vi "FIB realtime imaging PXIe-6124.vi"(0 "HW Config":T4={"FIB X coil"="FIB/ao0", "FIB Y coil"="FIB/ao1", "Beam blank"="FIB/port0/line0", "Ext Scan"="FIB/port0/line1", "Detector"="FIB/ai1", "Shutter Drive"="PXI1Slot2/ao0"}, 1 "Options":T3 {"Scan mode" items=["Raster", "Serpentine"]; "Det" items=["Detector A", "Detector B"]}, 2 "Single scan":bool, 3 "Scan Para":T2={"X resolution"=512, "Z resolution"=512, "X center"=0.0, "Z center"=0.0, "X size (V)"=10.0, "Z size (V)"=10.0, "Frame line rampdown ratio"=-0.1, "Scan rate (Hz)"=2000000, "Oversampling"=2} {"Frame line rampdown ratio" min=-1.0 max=1.0 step=0.05 format="%.2g"; "Scan rate (Hz)" max=4000000 format="%#.6p"}, 4 "As subVi":bool, 5 "COM port":refnum<visa-resource-name>="COM1", 6 "ActiveX Container":refnum<k7>(container)) -> (7 "Info & Status":T1={"Actual scan rate"=2000000.0, "X resolution with rampdown"=552, "Actual sample rate"=4000000.0, "Fetch backlog"=664878.0, "Total scan points"=276000, "Frame rate (/s)"=7} {"Fetch backlog" format="%#_6p"; "Actual sample rate" format="%#_6p"; "Actual scan rate" format="%#_4p"}, 10 "error out":errorcluster)   [LabVIEW 2018]
uses:
  <vilib>/DAQmx/write.llb/DAQmx Write (Analog 1D DBL NChan 1Samp).vi
  <vilib>/DAQmx/write.llb/DAQmx Write (Digital Wfm 1Chan NSamp).vi
  <vilib>/DAQmx/write.llb/DAQmx Write (Analog 2D DBL NChan NSamp).vi
  <vilib>/DAQmx/read.llb/DAQmx Read (Raw 1D I16).vi
  <vilib>/Analysis/2dsp.llb/Decimate (single shot, DBL).vi
  <vilib>/DAQmx/create/channels.llb/DAQmx Create Channel (AI-Voltage-Basic).vi
  <vilib>/DAQmx/create/channels.llb/DAQmx Create Channel (AO-Voltage-Basic).vi
  <vilib>/DAQmx/miscellaneous.llb/DAQmx Fill In Error Info.vi
  <vilib>/Waveform/DWDTOps.llb/DWDT Invert Digital.vi
  <vilib>/DAQmx/configure/timing.llb/DAQmx Timing (Sample Clock).vi
  <vilib>/DAQmx/create/channels.llb/DAQmx Create Channel (DO-Digital Output).vi
  <vilib>/DAQmx/create/channels.llb/DAQmx Create Channel (CO-Pulse Generation-Frequency).vi
  <vilib>/DAQmx/configure/trigger.llb/DAQmx Start Trigger (Digital Edge).vi
  <vilib>/Waveform/DWDTOps.llb/DWDT Uncompress Digital.vi
  <vilib>/Waveform/DWDTOps.llb/Digital Pattern Generator (Single Value).vi
  <vilib>/Analysis/NI_AALPro.lvlib
  <resource>/objmgr/daqmx.rc
panel:
  in  "Spot":bool
  out "Image shift":u32
  out "AI SampleClk.MaxRate":dbl
  in  "Sweep enabled":bool
  in  "Focus (V)":dbl min=-10.0 max=10.0 step=0.1 format="%.3g"
  in  "Sweep rate (Hz)":dbl=0.5 min=0.01 step=0.1 format="%0.2f"
  in  "Level #":u8
  in  "Sweep direction":bool
  in  "Angle (V)":dbl min=-10.0 max=10.0 step=0.1 format="%.3g"
  in  "Position (V)":dbl min=-10.0 max=10.0 step=0.1 format="%.3g"
  in  "Imbalance (V)":dbl min=-10.0 max=10.0 step=0.1 format="%.3f"
  out "Shutter Drive":tag
  out "Low blanked":bool
  in  "Machine Type":u8(ring) items=["Feiss", "NVision", "Jeiss"]
  out "Ext scan":tag
  out "Detector":tag="PXI1Slot7/ai0"
  out "FIB Y coil":tag="PXI1Slot7/ao1"
  out "FIB X coil":tag="PXI1Slot7/ao0"
  in  "Beam blanked":bool
  out "Beam blank":tag="PXI1Slot7/port0/line0"
  out "Oversampling":u16=2
  out "Scan rate (Hz)":u32=2000000
  out "Frame line rampdown ratio":dbl=0.1
  out "Y end":dbl=1.0
  out "X end":dbl=1.0
  out "Y start":dbl=-1.0
  out "X start":dbl=-1.0
  out "Y resolution":u32=500
  out "X resolution":u32=500
  out "Flip z":bool
  out "Flip x":bool
  out "Scan mode":u16
  out "Live image":i16[][](graph)
  in  "stop":bool=TRUE
  # "Flip"
  # "Scan coils"
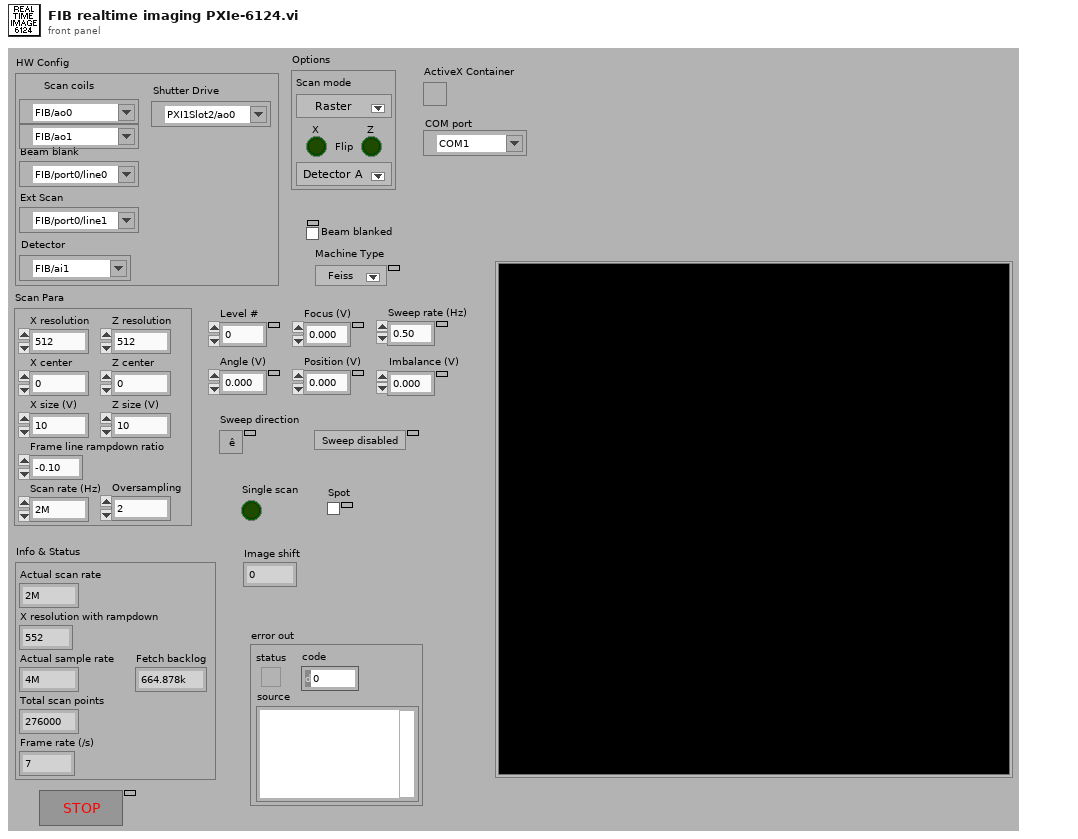
[diagram p1: front panel]
types:
  T1 = cluster{"Actual scan rate":dbl, "X resolution with rampdown":i32, "Actual sample rate":dbl, "Fetch backlog":dbl, "Total scan points":i32, "Frame rate (/s)":u32}
  T2 = cluster{"X resolution":u32, "Z resolution":u32, "X center":dbl, "Z center":dbl, "X size (V)":dbl, "Z size (V)":dbl, "Frame line rampdown ratio":dbl, "Scan rate (Hz)":u32, "Oversampling":u16}
  T3 = cluster{"Scan mode":u16, "Flip x":bool, "Flip z":bool, "Det":u16}
  T4 = cluster{"FIB X coil":tag, "FIB Y coil":tag, "Beam blank":tag, "Ext Scan":tag, "Detector":tag, "Shutter Drive":tag}
  T5 = enum16{"SEM", "FIB", "Milling", "SEM + FIB", "Mill + SEM", "SEM Drift Correction", "FIB Drift Correction", "No Beam", "External", "External + SEM"}
  T6 = enum16{"SEM", "FIB", "Mill", "SEM + FIB", "Mill + SEM", "Drift SEM", "Drift FIB", "None", "Ext", "Ext + SEM"}
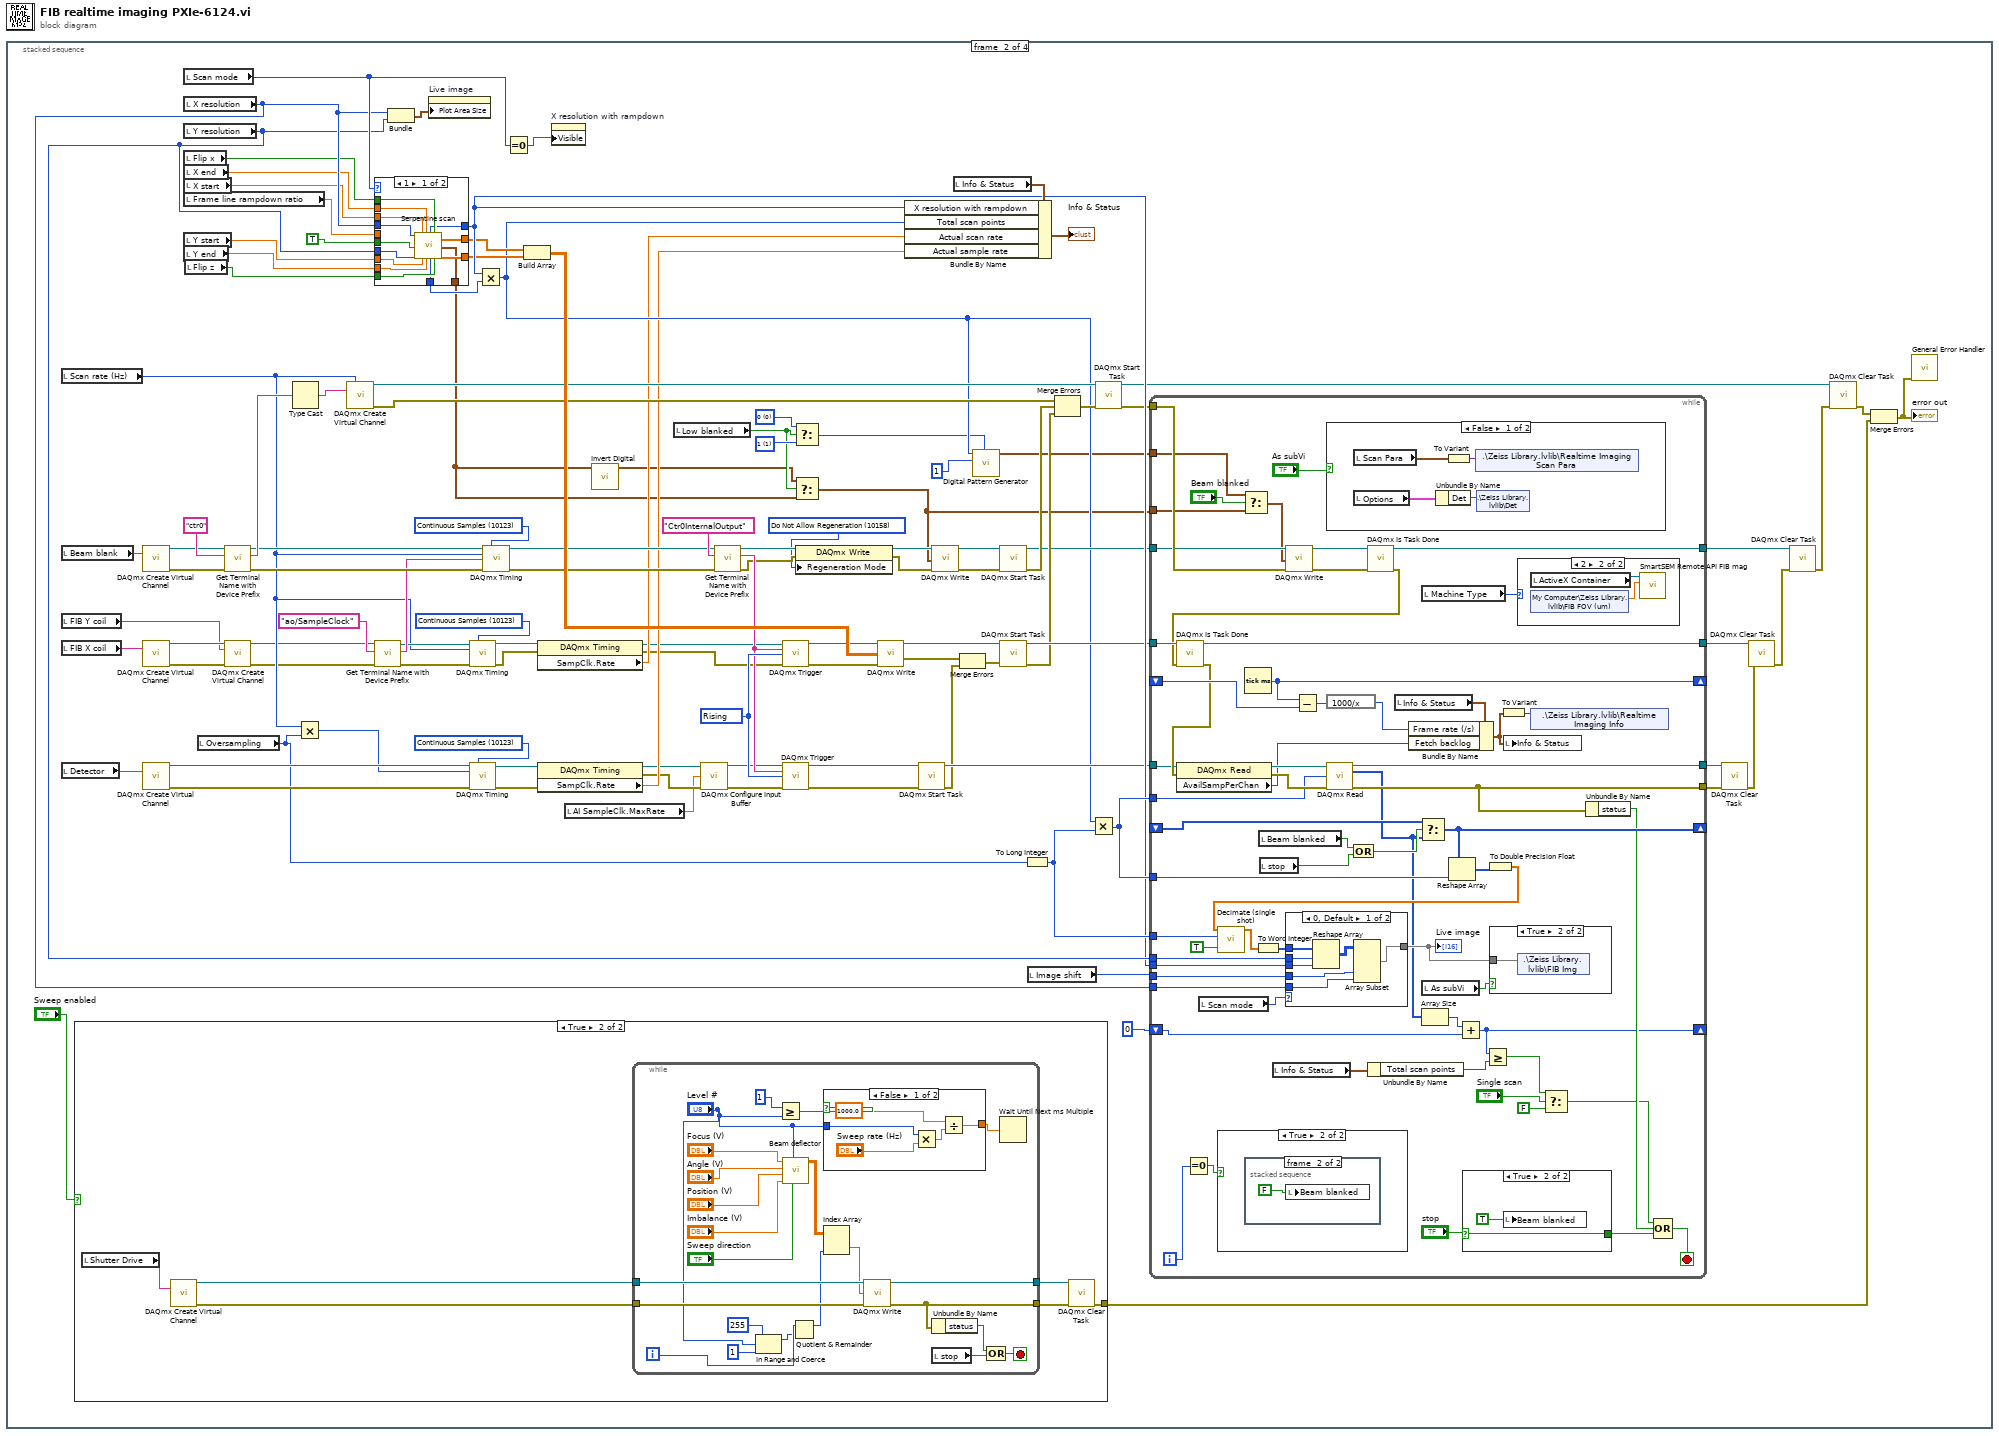
[diagram p0: block diagram]
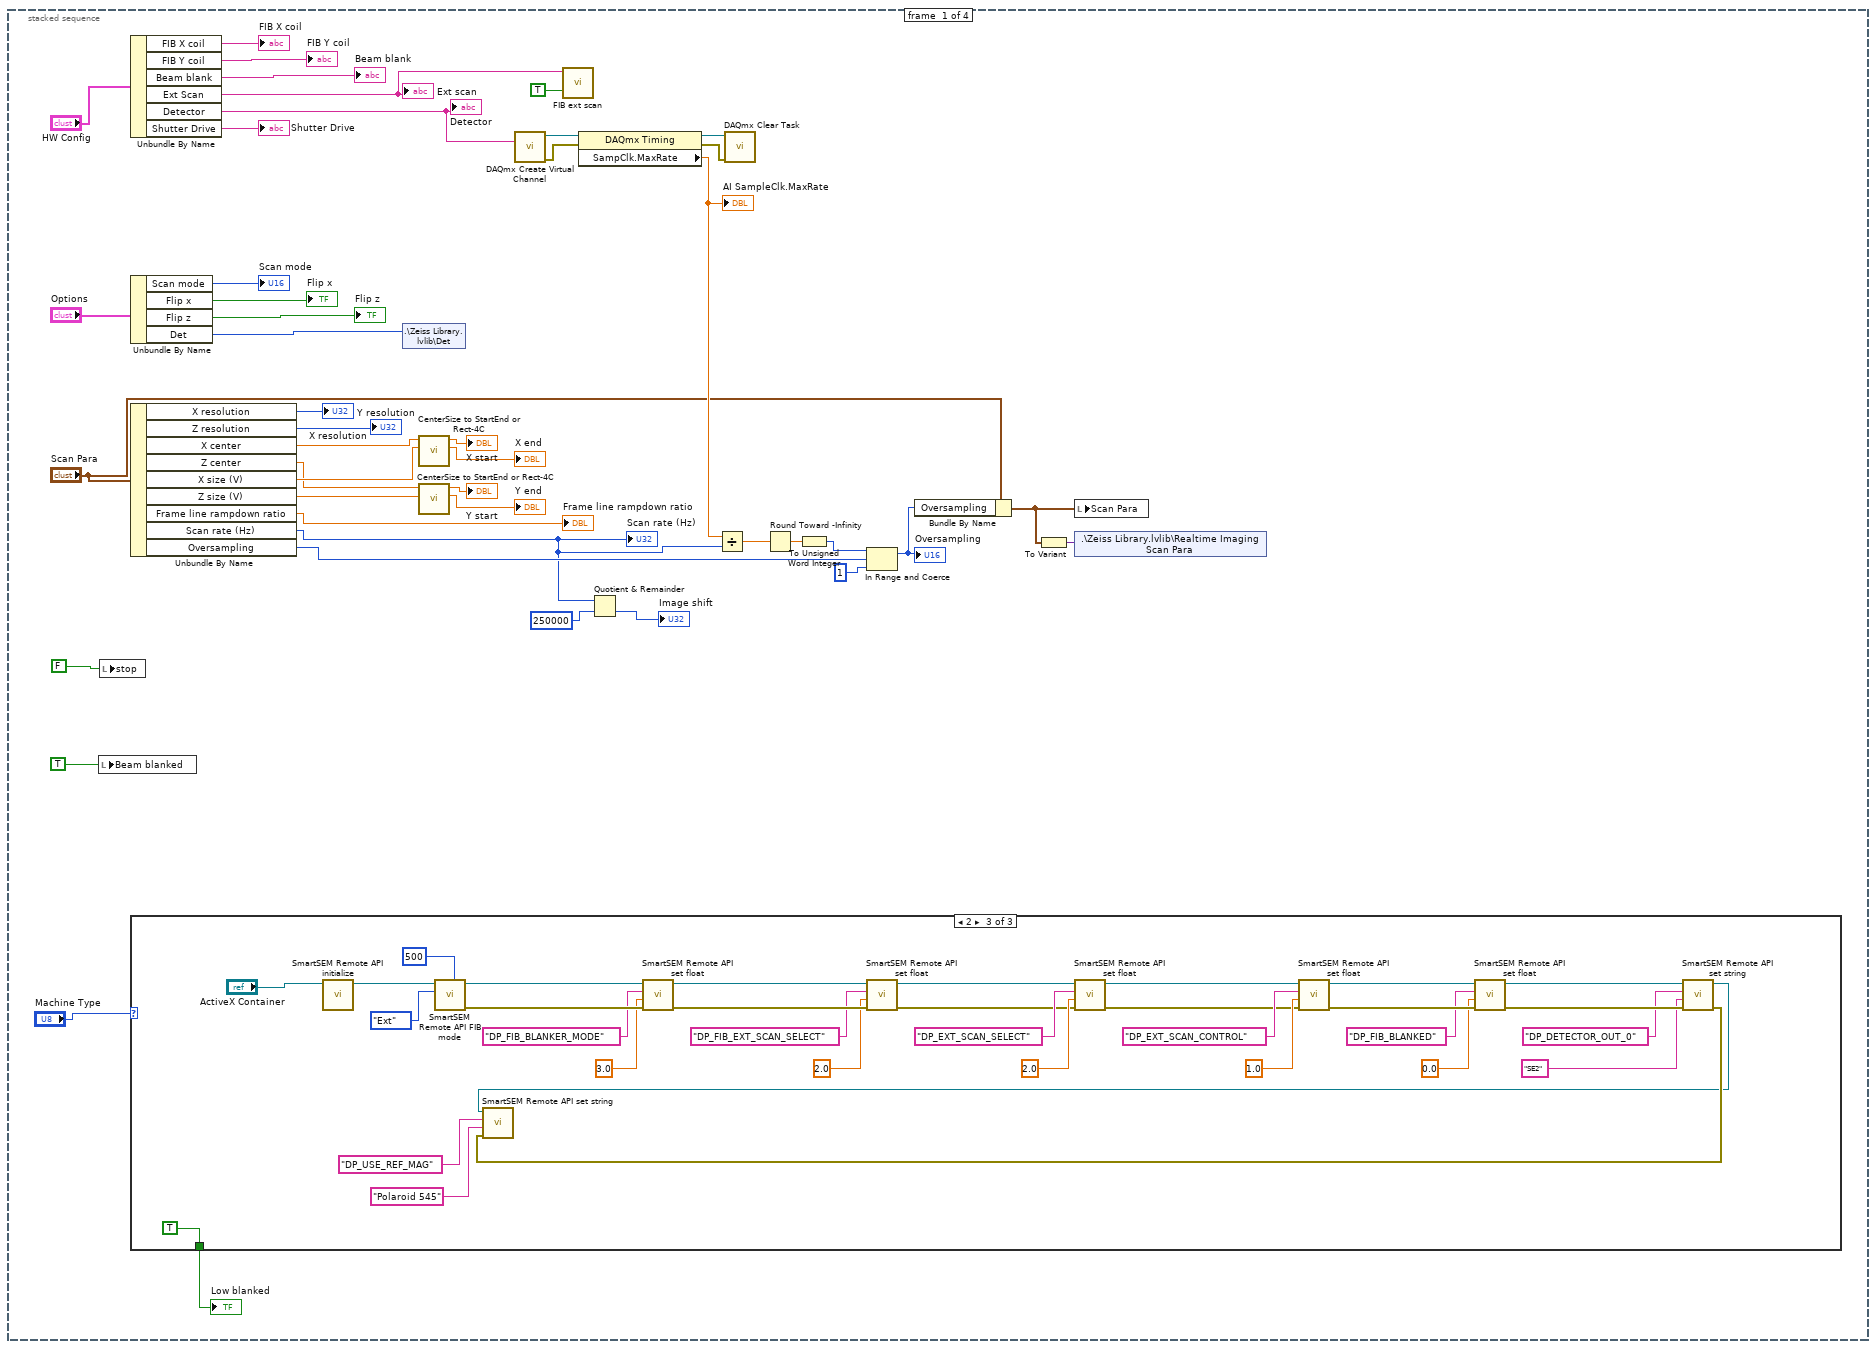
[diagram p2: hidden frame]
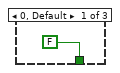
[diagram p3: hidden frame]
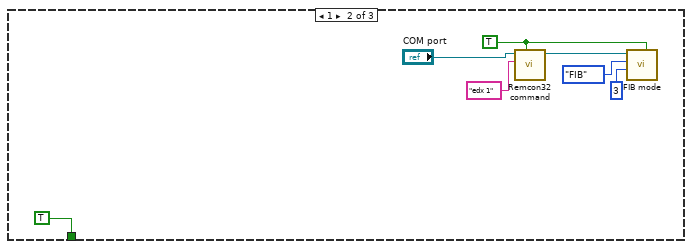
[diagram p4: hidden frame]
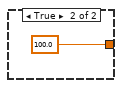
[diagram p6: hidden frame]
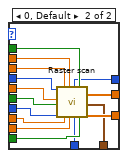
[diagram p7: hidden frame]
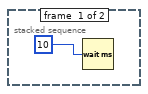
[diagram p11: hidden frame]
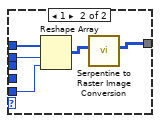
[diagram p14: hidden frame]
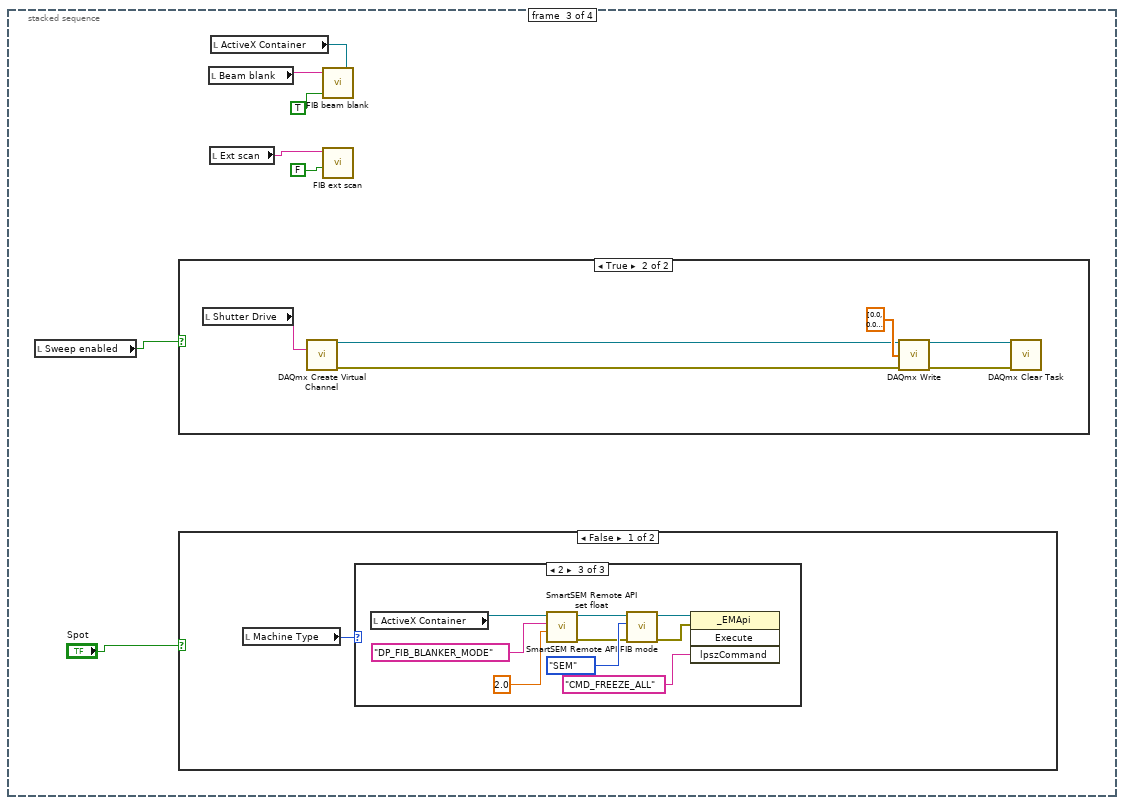
[diagram p15: hidden frame]
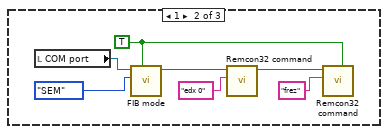
[diagram p17: hidden frame]
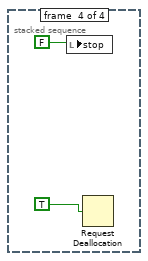
[diagram p20: hidden frame]
diagram:
  n1 = stacked-sequence {
    frame #0 {
      n2 = local write "Beam blanked"(TRUE ("Beam blanked")) -> ()
      n3 = local write "stop"(FALSE ("stop")) -> ()
      n4 = Unbundle By Name("HW Config") -> ("FIB X coil"=→"FIB X coil":tag, "FIB Y coil"=→"FIB Y coil":tag, "Beam blank"=→"Beam blank":tag, "Ext Scan"=w23:tag, "Detector"=w16:tag, "Shutter Drive"=→"Shutter Drive":tag)
      "Detector" <- w16
      "Ext scan" <- w23
      n5 = Unbundle By Name("Options") -> ("Scan mode"=→"Scan mode":u16, "Flip x"=→"Flip x":bool, "Flip z"=→"Flip z":bool, "Det"=w37:u16)
      n6 = Unbundle By Name("Scan Para") -> ("X resolution"=→"X resolution":u32, "Z resolution"=→"Y resolution":u32, "X center"=w34:dbl, "Z center"=w30:dbl, "X size (V)"=w33:dbl, "Z size (V)"=w29:dbl, "Frame line rampdown ratio"=→"Frame line rampdown ratio":dbl, "Scan rate (Hz)"=w5:u32, "Oversampling"=w15:u16)
      "Scan rate (Hz)" <- w5
      n7 = case shown="2" "Machine Type" {
        tunnel: [FALSE ("Beam blanked") TRUE ("Beam blanked") TRUE ("Beam blanked")] -> w21
        frame 0, Default {
        }
        frame 1 {
          w50 = TRUE ("Close session")
          n8 = call "Remcon32 command.vi"("Initialization"=w50, "SEM command"="edx 1", "COM port in"="COM port") -> ("COM port out"=w49:refnum<visa-resource-name>)  [unwired: 5 in, 3 out]
          n9 = call "FIB mode.vi"("Close session"=w50, "Iterations"=u32 3, "FIB mode"=T5."FIB", "COM port in"=w49) -> ()  [unwired: 6 in, 2 out]
        }
        frame 2 {
          n10 = call "SmartSEM Remote API initialize.vi"("ActiveX Container"="ActiveX Container") -> ("reference out"=w58:refnum<k7>)  [unwired: 9 in, 1 out]
          n11 = call "SmartSEM Remote API FIB mode.vi"("Wait (ms)"=u32 500, "FIB mode"=T6."Ext", "ActiveX Container"=w58) -> ("error out"=w83:errorcluster, "reference out"=w84:refnum<k7>)  [unwired: 7 in]
          n12 = call "SmartSEM Remote API set float.vi"("error in"=w83, "vValue"=sgl 3.0, "lpszParam"="DP_FIB_BLANKER_MODE", "ActiveX Container"=w84) -> ("error out"=w79:errorcluster, "reference out"=w80:refnum<k7>)  [unwired: 6 in]
          n13 = call "SmartSEM Remote API set float.vi"("error in"=w79, "vValue"=sgl 2.0, "lpszParam"="DP_FIB_EXT_SCAN_SELECT" ("lpszCommand"), "ActiveX Container"=w80) -> ("error out"=w57:errorcluster, "reference out"=w55:refnum<k7>)  [unwired: 6 in]
          n14 = call "SmartSEM Remote API set float.vi"("error in"=w57, "vValue"=sgl 2.0, "lpszParam"="DP_EXT_SCAN_SELECT" ("lpszCommand"), "ActiveX Container"=w55) -> ("error out"=w56:errorcluster, "reference out"=w54:refnum<k7>)  [unwired: 6 in]
          n15 = call "SmartSEM Remote API set float.vi"("error in"=w56, "vValue"=sgl 1.0, "lpszParam"="DP_EXT_SCAN_CONTROL" ("lpszCommand"), "ActiveX Container"=w54) -> ("error out"=w73:errorcluster, "reference out"=w74:refnum<k7>)  [unwired: 6 in]
          n16 = call "SmartSEM Remote API set float.vi"("error in"=w73, "vValue"=sgl 0.0, "lpszParam"="DP_FIB_BLANKED", "ActiveX Container"=w74) -> ("error out"=w69:errorcluster, "reference out"=w70:refnum<k7>)  [unwired: 6 in]
          n17 = call "SmartSEM Remote API set string.vi"("error in"=w69, "vValue"="SE2" ("Det A Type"), "lpszParam"="DP_DETECTOR_OUT_0", "ActiveX Container"=w70) -> ("error out"=w61:errorcluster, "reference out"=w60:refnum<k7>)  [unwired: 6 in]
          n18 = call "SmartSEM Remote API set string.vi"("error in"=w61, "vValue"="Polaroid 545" ("lpszParam"), "lpszParam"="DP_USE_REF_MAG", "ActiveX Container"=w60) -> ()  [unwired: 6 in, 2 out]
        }
      }
      "Low blanked" <- w21
      n19 = shared-variable ".\\Zeiss Library.lvlib\\Det"(w37) -> ()  [unwired: 1 in, 1 out]
      n20 = call "CenterSize to StartEnd or Rect-4C.vi"("Size"=w33, "Center"=w34) -> ("End"=→"X end":dbl, "Start"=→"X start":dbl)  [unwired: 3 in, 1 out]
      n21 = call "CenterSize to StartEnd or Rect-4C.vi"("Size"=w29, "Center"=w30) -> ("End"=→"Y end":dbl, "Start"=→"Y start":dbl)  [unwired: 3 in, 1 out]
      n22 = call-poly <vilib>:"DAQmx Create Virtual Channel.vi"("physical channels"=w16) -> ("task out"=w18:refnum<k21>, "error out"=w20:errorcluster)  [unwired: 8 in, 5 out]
      n23 = call "FIB ext scan.vi"("Ext on"=TRUE ("data"), "FIB Ext Scan"=w23) -> ()  [unwired: 9 in, 1 out]
      n24 = property class="DAQmx Timing"(reference=w18, error in=w20) -> (reference out=w17:refnum<k21>, error out=w19:errorcluster, "SampClk.MaxRate"=w13:dbl)
      "AI SampleClk.MaxRate" <- w13
      n25 = Quotient & Remainder(x=w5, y=u32 250000) -> (floor(x/y)=→"Image shift":u32)  [unwired: 1 out]
      n26 = Divide(x=w13, y=w5) -> (x/y=w12:dbl)
      n27 = call <vilib>:"DAQmx Clear Task.vi"("task in"=w17, "error in"=w19) -> ()  [unwired: 14 out]
      n28 = Round Toward -Infinity(1:w12) -> (0:w11:dbl)
      n29 = To Unsigned Word Integer(number=w11) -> (unsigned 16bit integer=w10:u16)
      n30 = In Range and Coerce(upper limit=w10, x=w15, lower limit=u16 1) -> (coerced(x)=w8:u16)  [unwired: 1 out]
      "Oversampling" <- w8
      n31 = Bundle By Name(cluster="Scan Para", "Oversampling"=w8) -> (w7:T2)
      n32 = To Variant(anything=w7) -> (Variant=w36:variant)
      n33 = local write "Scan Para"(w7) -> ()
      n34 = shared-variable ".\\Zeiss Library.lvlib\\Realtime Imaging Scan Para"(w36) -> ()  [unwired: 1 in, 1 out]
    }
    frame #1 {
      w105 = u8 1 items=["0", "1", "Z", "L", "H", "X", "T", "V"] ("value")
      w106 = u8 0 items=["0", "1", "Z", "L", "H", "X", "T", "V"] ("value")
      w117 = 10158 items=["Allow Regeneration"=10097, "Do Not Allow Regeneration"=10158] ("RegenMode")
      w142 = 10123 items=["Finite Samples"=10178, "Continuous Samples"=10123] ("sample mode")
      w130 = 10280 items=["Rising"=10280, "Falling"=10171] ("edge")
      w173 = 10123 items=["Finite Samples"=10178, "Continuous Samples"=10123, "Hardware Timed Single Point"=12522] ("sample mode")
      w177 = 10123 items=["Finite Samples"=10178, "Continuous Samples"=10123, "Hardware Timed Single Point"=12522] ("sample mode")
      n35 = local read "Scan rate (Hz)"() -> (w123:u32)
      n36 = local read "Beam blank"() -> (w111:tag)
      n37 = local read "FIB Y coil"() -> (w178:tag)
      n38 = local read "FIB X coil"() -> (w179:tag)
      n39 = local read "Detector"() -> (w180:tag)
      n40 = case shown="True" "Sweep enabled" {
        tunnel: [_ w207] -> w99
        frame False {
        }
        frame True {
          n41 = local read "Shutter Drive"() -> (w206:tag)
          n42 = call-poly <vilib>:"DAQmx Create Virtual Channel.vi"("physical channels"=w206) -> ("task out"=w203:refnum<k21>, "error out"=w202:errorcluster)  [unwired: 13 in]
          n43 = while {
            tunnel: [w226] -> w205
            tunnel: [w227] -> w204
            tunnel: w203 -> [w225]
            tunnel: w202 -> [w224]
            i -> [w222]
            stop <- w230 stop-if-true
            n44 = In Range and Coerce(upper limit=u8 255 ("lower limit"), x="Level #", lower limit=u8 1) -> (coerced(x)=w216:u8)  [unwired: 1 out]
            n45 = Greater Or Equal?(x=u8 1 ("y"), y="Level #") -> (x >= y?=w220:bool)
            n46 = call "Beam deflector.vi"("Sweep direction"="Sweep direction", "Level #"="Level #", "Imbalance (V)"="Imbalance (V)", "Position (V)"="Position (V)", "Angle (V)"="Angle (V)", "Focus (V)"="Focus (V)") -> ("All posts"=w209:dbl[][])  [unwired: 5 in]
            n47 = Quotient & Remainder(x=w222, y=w216) -> (x-y*floor(x/y)=w219:i32)  [unwired: 1 out]
            n48 = case shown="False" w220 {
              tunnel: "Level #" -> [w234 _]
              tunnel: [w231 100.0] -> w221
              frame False {
                n49 = Multiply(x=w234, y="Sweep rate (Hz)") -> (x*y=w233:dbl)
                n50 = Divide(x=1000.0, y=w233) -> (x/y=w231:dbl)
              }
              frame True {
              }
            }
            n51 = Index Array(array=w209, index (col)=w219) -> (element=w208:dbl[])  [unwired: 1 in]
            n52 = call-poly <vilib>:"DAQmx Write.vi"("task/channels in"=w225, "data"=w208, "error in"=w224) -> ("task out"=w227:refnum<k21>, "error out"=w226:errorcluster)  [unwired: 1 in, 10 out]
            n53 = Unbundle By Name(w226) -> ("status"=w228:bool)
            n54 = local read "stop"() -> (w229:bool)
            n55 = Compound Arithmetic op=OR(w228, w229) -> (w230:bool)
            n56 = Wait Until Next ms Multiple(millisecond multiple=w221) -> ()  [unwired: 1 out]
          }
          n57 = call <vilib>:"DAQmx Clear Task.vi"("task in"=w204, "error in"=w205) -> ("error out"=w207:errorcluster)  [unwired: 13 in]
        }
      }
      n58 = call-poly <vilib>:"DAQmx Create Virtual Channel.vi"("lines"=w111) -> ("task out"=w149:refnum<k21>, "error out"=w151:errorcluster)  [unwired: 6 in, 7 out]
      n59 = call-poly <vilib>:"DAQmx Create Virtual Channel.vi"("physical channels"=w179) -> ("task out"=w182:refnum<k21>, "error out"=w181:errorcluster)  [unwired: 8 in, 5 out]
      n60 = call-poly <vilib>:"DAQmx Create Virtual Channel.vi"("physical channels"=w180) -> ("task out"=w175:refnum<k21>, "error out"=w174:errorcluster)  [unwired: 8 in, 5 out]
      n61 = local read "Scan mode"() -> (w198:u16)
      n62 = local read "X resolution"() -> (w197:u32)
      n63 = local read "Y resolution"() -> (w196:u32)
      n64 = local read "Flip x"() -> (w188:bool)
      n65 = local read "X end"() -> (w185:dbl)
      n66 = local read "X start"() -> (w186:dbl)
      n67 = local read "Frame line rampdown ratio"() -> (w195:dbl)
      n68 = local read "Y start"() -> (w184:dbl)
      n69 = local read "Y end"() -> (w183:dbl)
      n70 = local read "Flip z"() -> (w187:bool)
      n71 = local read "Oversampling"() -> (w122:u16)
      n72 = call "Get Terminal Name with Device Prefix.vi"("error in"=w151, "Local Terminal Name"="ctr0", "task/channels in"=w149) -> ("error out"=w152:errorcluster, "Terminal Name with Device Prefix"=w154:tag, "task out"=w150:refnum<k21>)  [unwired: 6 in]
      n73 = call-poly <vilib>:"DAQmx Create Virtual Channel.vi"("task in"=w182, "physical channels"=w178, "error in"=w181) -> ("task out"=w90:refnum<k21>, "error out"=w89:errorcluster)  [unwired: 6 in, 5 out]
      n74 = Type Cast(x=w154) -> (*(type *) &x=w155:string)  [unwired: 1 in]
      n75 = Multiply(x=w123, y=w122) -> (x*y=w124:u32)
      n76 = call-poly <vilib>:"DAQmx Create Virtual Channel.vi"("frequency"=w123, "counter"=w155) -> ("task out"=w145:refnum<k21>, "error out"=w147:errorcluster)  [unwired: 7 in, 5 out]
      n77 = case shown="1" w198 {
        tunnel: w195 -> [_ w262]
        tunnel: w188 -> [w245 w265]
        tunnel: w196 -> [w248 w260]
        tunnel: w197 -> [w250 w263]
        tunnel: w187 -> [w242 w264]
        tunnel: [w241 w259] -> w191
        tunnel: [w240 w258] -> w190
        tunnel: TRUE ("Flip x") -> [w249 w261]
        tunnel: w186 -> [w247 w257]
        tunnel: w185 -> [w246 w256]
        tunnel: w184 -> [w244 w255]
        tunnel: w183 -> [w243 w254]
        tunnel: [w239 w253] -> w168
        tunnel: [w238 w252] -> w167
        tunnel: [w237 w251] -> w91
        frame 1 {
          n78 = call "Serpentine scan.vi"("X resolution"=w250, "Scan pattern?"=w249, "Y resolution"=w248, "X start"=w247, "Y start"=w244, "X end"=w246, "Y end"=w243, "Flip x"=w245, "Flip y"=w242) -> ("X resolution with rampdown"=w241:i32, "Y resolution"=w240:i32, "X scan pattern"=w239:dbl[], "Blanking pattern"=w237:digitalwaveform, "Y scan pattern"=w238:dbl[])  [unwired: 3 in, 3 out]
        }
        frame 0, Default {
          n79 = call "Raster scan.vi"("X resolution"=w263, "Frame line rampdown ratio"=w262, "Scan pattern?"=w261, "Y resolution"=w260, "X start"=w257, "Y start"=w255, "X end"=w256, "Y end"=w254, "Flip x"=w265, "Flip y"=w264) -> ("X resolution with rampdown"=w259:i32, "Y resolution"=w258:i32, "X scan pattern"=w253:dbl[], "Blanking pattern"=w251:digitalwaveform, "Y scan pattern"=w252:dbl[])  [unwired: 2 in, 3 out]
        }
      }
      n80 = call "Get Terminal Name with Device Prefix.vi"("error in"=w89, "Local Terminal Name"="ao/SampleClock", "task/channels in"=w90) -> ("error out"=w125:errorcluster, "Terminal Name with Device Prefix"=w138:tag, "task out"=w126:refnum<k21>)  [unwired: 6 in]
      n81 = Bundle("X resolution"=w197, "Y resolution"=w196) -> (w200:cluster{"X resolution":u32, "Y resolution":u32})  [unwired: 1 in]
      n82 = property on="Live image" class="IntGraph (strict)"("Plot Area Size"=w200) -> ()  [unwired: 2 in, 2 out]
      n83 = call-poly <vilib>:"DAQmx Timing.vi"("task/channels in"=w126, "sample mode"=w177, "rate"=w123, "error in"=w125) -> ("task out"=w128:refnum<k21>, "error out"=w127:errorcluster)  [unwired: 3 in, 7 out]
      n84 = call-poly <vilib>:"DAQmx Timing.vi"("task/channels in"=w175, "sample mode"=w173, "rate"=w124, "error in"=w174) -> ("task out"=w172:refnum<k21>, "error out"=w171:errorcluster)  [unwired: 3 in, 7 out]
      n85 = Multiply(x=w191, y=w190) -> (x*y=w115:i32)
      n86 = call-poly <vilib>:"DAQmx Timing.vi"("task/channels in"=w150, "sample mode"=w142, "rate"=w123, "source"=w138, "error in"=w152) -> ("task out"=w141:refnum<k21>, "error out"=w140:errorcluster)  [unwired: 2 in, 7 out]
      n87 = Equal To 0?(x=w198) -> (x = 0?=w192:bool)
      n88 = Build Array(w168, w167) -> (w166:dbl[][])
      n89 = property class="DAQmx Timing"(reference=w128, error in=w127) -> (reference out=w108:refnum<k21>, error out=w107:errorcluster, "SampClk.Rate"=w110:dbl)
      n90 = property class="DAQmx Timing"(reference=w172, error in=w171) -> (reference out=w97:refnum<k21>, error out=w94:errorcluster, "SampClk.Rate"=w109:dbl)
      n91 = property on="X resolution with rampdown" class="DigNum (strict)"("Visible"=w192) -> ()  [unwired: 2 in, 2 out]
      n92 = local read "AI SampleClk.MaxRate"() -> (w93:dbl)
      n93 = call-poly <vilib>:"Invert Digital.vi"("digital waveform"=w91) -> ("inverted waveform"=w92:digitalwaveform)  [unwired: 9 in, 1 out]
      n94 = local read "Low blanked"() -> (w102:bool)
      n95 = call <vilib>:"DAQmx Configure Input Buffer.vi"("task/channels in"=w97, "buffer size (in samples per channel)"=w93, "error in"=w94) -> ("task out"=w96:refnum<k21>, "error out"=w95:errorcluster)  [unwired: 11 in]
      n96 = call "Get Terminal Name with Device Prefix.vi"("error in"=w140, "Local Terminal Name"="Ctr0InternalOutput" ("terminal"), "task/channels in"=w141) -> ("error out"=w119:errorcluster, "Terminal Name with Device Prefix"=w129:tag, "task out"=w121:refnum<k21>)  [unwired: 1 in, 5 out]
      n97 = call-poly <vilib>:"DAQmx Trigger.vi"("task/channels in"=w108, "source"=w129, "edge"=w130, "error in"=w107) -> ("task out"=w131:refnum<k21>, "error out"=w132:errorcluster)  [unwired: 10 out]
      n98 = call-poly <vilib>:"DAQmx Trigger.vi"("task/channels in"=w96, "source"=w129, "edge"=w130, "error in"=w95) -> ("task out"=w170:refnum<k21>, "error out"=w169:errorcluster)  [unwired: 10 out]
      n99 = Select(t=w106, s=w102, f=w105) -> (s? t:f=w104:u8)
      n100 = Select(t=w92, s=w102, f=w91) -> (s? t:f=w103:digitalwaveform)
      n101 = property class="DAQmx Write"(reference=w121, error in=w119, "Regeneration Mode"=w117) -> (reference out=w120:refnum<k21>, error out=w118:errorcluster)
      n102 = call-poly <vilib>:"DAQmx Write.vi"("task/channels in"=w131, "data"=w166, "error in"=w132) -> ("task out"=w165:refnum<k21>, "error out"=w163:errorcluster)  [unwired: 1 in, 10 out]
      n103 = call <vilib>:"DAQmx Start Task.vi"("task/channels in"=w170, "error in"=w169) -> ("task out"=w162:refnum<k21>, "error out"=w161:errorcluster)  [unwired: 12 out]
      n104 = call-poly <vilib>:"DAQmx Write.vi"("task/channels in"=w120, "data"=w103, "error in"=w118) -> ("task out"=w144:refnum<k21>, "error out"=w139:errorcluster)  [unwired: 2 in, 9 out]
      n105 = local read "Info & Status"() -> (w194:T1)
      n106 = Bundle By Name(cluster=w194, "X resolution with rampdown"=w191, "Total scan points"=w115, "Actual scan rate"=w110, "Actual sample rate"=w109) -> (→"Info & Status":T1)
      n107 = Merge Errors(w163, w161) -> (w164:errorcluster)
      n108 = call-poly <vilib>:"Digital Pattern Generator.vi"("value"=w104, "number of signals"=u32 1, "number of samples"=w115) -> ("digital waveform"=w114:digitalwaveform)  [unwired: 2 in, 6 out]
      n109 = call <vilib>:"DAQmx Start Task.vi"("task/channels in"=w144, "error in"=w139) -> ("task out"=w135:refnum<k21>, "error out"=w146:errorcluster)  [unwired: 12 out]
      n110 = call <vilib>:"DAQmx Start Task.vi"("task/channels in"=w165, "error in"=w164) -> ("task out"=w160:refnum<k21>, "error out"=w137:errorcluster)  [unwired: 12 out]
      n111 = To Long Integer(number=w122) -> (32bit integer=w201:i32)
      n112 = local read "Image shift"() -> (w87:u32)
      n113 = Merge Errors(w147, w146, w137) -> (w148:errorcluster)
      n114 = Multiply(x=w115, y=w201) -> (x*y=w199:i32)
      n115 = call <vilib>:"DAQmx Start Task.vi"("task/channels in"=w145, "error in"=w148) -> ("task out"=w134:refnum<k21>, "error out"=w136:errorcluster)  [unwired: 12 out]
      n116 = while {
        shift-right: [w323] -> _
        shift-left: _ -> [w322]
        tunnel: w201 -> [w321]
        tunnel: w196 -> [w320]
        tunnel: w191 -> [w319]
        tunnel: w197 -> [w318]
        tunnel: w199 -> [w289]
        tunnel: w199 -> [w317]
        shift-right: [w300] -> _
        shift-left: _ -> [w308]
        tunnel: w162 -> [w291]
        tunnel: w160 -> [w299]
        tunnel: [w298] -> w158
        tunnel: [w297] -> w159
        tunnel: [w296] -> w157
        tunnel: w136 -> [w284]
        tunnel: w135 -> [w283]
        tunnel: [w287] -> w133
        tunnel: w103 -> [w281]
        tunnel: w114 -> [w280]
        shift-right: [w274] -> _
        shift-left: 0 -> [w276]
        tunnel: w87 -> [w267]
        i -> [w301]
        stop <- w329 stop-if-true
        n117 = Equal To 0?(x=w301) -> (x = 0?=w302:bool)
        n118 = local read "Scan mode"() -> (w316:u16)
        n119 = case shown="True" w302 {
          frame False {
          }
          frame True {
            n120 = stacked-sequence {
              frame #0 {
                n121 = Wait (ms)(milliseconds to wait=u32 10) -> ()  [unwired: 1 out]
              }
              frame #1 {
                n122 = local write "Beam blanked"(FALSE ("Beam blanked")) -> ()
              }
            }
          }
        }
        n123 = Select(t=w280, s="Beam blanked", f=w281) -> (s? t:f=w268:digitalwaveform)
        n124 = Tick Count (ms)() -> (millisecond timer value=w323:u32)
        n125 = local read "Beam blanked"() -> (w305:bool)
        n126 = local read "stop"() -> (w303:bool)
        n127 = local read "Info & Status"() -> (w275:T1)
        n128 = call-poly <vilib>:"DAQmx Write.vi"("task/channels in"=w283, "data"=w268, "error in"=w284) -> ("task out"=w282:refnum<k21>, "error out"=w285:errorcluster)  [unwired: 2 in, 9 out]
        n129 = Subtract(x=w323, y=w322) -> (x-y=w310:u32)
        n130 = case shown="False" "As subVi" {
          frame False {
            n131 = local read "Scan Para"() -> (w332:T2)
            n132 = local read "Options"() -> (w335:T3)
            n133 = Unbundle By Name(w335) -> ("Det"=w334:u16)
            n134 = To Variant(anything=w332) -> (Variant=w333:variant)
            n135 = shared-variable ".\\Zeiss Library.lvlib\\Realtime Imaging Scan Para"(w333) -> ()  [unwired: 1 in, 1 out]
            n136 = shared-variable ".\\Zeiss Library.lvlib\\Det"(w334) -> ()  [unwired: 1 in, 1 out]
          }
          frame True {
          }
        }
        n137 = expression code="1000/x"(w310) -> (w313:u32)
        n138 = Compound Arithmetic op=OR(w305, w303) -> (w304:bool)
        n139 = call <vilib>:"DAQmx Is Task Done.vi"("task/channels in"=w282, "error in"=w285) -> ("task out"=w287:refnum<k21>, "error out"=w288:errorcluster)  [unwired: 2 in, 10 out]
        n140 = call <vilib>:"DAQmx Is Task Done.vi"("task/channels in"=w299, "error in"=w288) -> ("task out"=w296:refnum<k21>, "error out"=w294:errorcluster)  [unwired: 2 in, 10 out]
        n141 = property class="DAQmx Read"(reference=w291, error in=w294) -> (reference out=w292:refnum<k21>, error out=w293:errorcluster, "AvailSampPerChan"=w290:u32)
        n142 = call-poly <vilib>:"DAQmx Read.vi"("task/channels in"=w292, "number of samples per channel"=w289, "error in"=w293) -> ("task out"=w297:refnum<k21>, "data"=w278:i16[], "error out"=w298:errorcluster)  [unwired: 10 out]
        n143 = Unbundle By Name(w275) -> ("Total scan points"=w273:i32)
        n144 = local read "Info & Status"() -> (w314:T1)
        n145 = Bundle By Name(cluster=w314, "Frame rate (/s)"=w313, "Fetch backlog"=w290) -> (w311:T1)
        n146 = Select(t=w308, s=w304, f=w278) -> (s? t:f=w300:i16[])
        n147 = local read "Machine Type"() -> (w266:u8)
        n148 = local read "As subVi"() -> (w309:bool)
        n149 = Array Size(array=w278) -> (size(s)=w277:i32)
        n150 = Reshape Array(w300, w317) -> (w325:i16[])
        n151 = Add(x=w277, y=w276) -> (x+y=w274:i32)
        n152 = case shown="True" "stop" {
          selector: "stop" -> [w338 w340]
          tunnel: [w338 w340] -> w306
          frame False {
          }
          frame True {
            n153 = local write "Beam blanked"(TRUE ("Beam blanked")) -> ()
          }
        }
        n154 = Greater Or Equal?(x=w274, y=w273) -> (x >= y?=w271:bool)
        n155 = To Double Precision Float(number=w325) -> (double precision float=w324:dbl[])
        n156 = call-poly <vilib>:"Decimate (single shot).vi"("averaging"=TRUE, "decimating factor"=w321, "X"=w324) -> ("Decimated Array"=w327:dbl[])  [unwired: 8 out]
        n157 = To Word Integer(number=w327) -> (16bit integer=w326:i16[])
        n158 = case shown="0, Default" w316 {
          tunnel: w326 -> [w348 w353]
          tunnel: w320 -> [w346 w352]
          tunnel: w319 -> [w345 _]
          tunnel: w318 -> [w344 w351]
          tunnel: [w343 w349] -> w315
          tunnel: w267 -> [w342 _]
          frame 0, Default {
            n159 = Reshape Array(w348, w346, w345) -> (w347:i16[][])
            n160 = Array Subset(array=w347, index (col)=w342, length (col)=w344) -> (w343:i16[][])  [unwired: 2 in]
          }
          frame 1 {
            n161 = Reshape Array(w353, w352, w351) -> (w350:i16[][])
            n162 = call "Serpentine to Raster Image Conversion.vi"("Input"=w350) -> ("Output"=w349:i16[][])  [unwired: 10 in]
          }
        }
        "Live image" <- w315
        n163 = case shown="True" w309 {
          tunnel: w315 -> [_ w341]
          frame False {
          }
          frame True {
            n164 = shared-variable ".\\Zeiss Library.lvlib\\FIB Img"(w341) -> ()  [unwired: 1 in, 1 out]
          }
        }
        n165 = To Variant(anything=w311) -> (Variant=w312:variant)
        n166 = local write "Info & Status"(w311) -> ()
        n167 = case shown="2" w266 {
          frame 0, Default {
          }
          frame 2 {
            n168 = local read "ActiveX Container"() -> (w331:refnum<k7>)
            n169 = shared-variable "My Computer\\Zeiss Library.lvlib\\FIB FOV (um)"() -> (w330:sgl)  [unwired: 1 in, 1 out]
            n170 = call "SmartSEM Remote API FIB mag.vi"("FIB FOV (um)"=w330, "ActiveX Container"=w331) -> ()  [unwired: 8 in, 2 out]
          }
        }
        n171 = shared-variable ".\\Zeiss Library.lvlib\\Realtime Imaging Info"(w312) -> ()  [unwired: 1 in, 1 out]
        n172 = Select(t=w271, s="Single scan", f=FALSE) -> (s? t:f=w269:bool)
        n173 = Unbundle By Name(w298) -> ("status"=w295:bool)
        n174 = Compound Arithmetic op=OR(w269, w295, w306) -> (w329:bool)
      }
      n175 = call <vilib>:"DAQmx Clear Task.vi"("task in"=w159, "error in"=w158) -> ("error out"=w156:errorcluster)  [unwired: 13 out]
      n176 = call <vilib>:"DAQmx Clear Task.vi"("task in"=w157, "error in"=w156) -> ("error out"=w113:errorcluster)  [unwired: 13 out]
      n177 = call <vilib>:"DAQmx Clear Task.vi"("task in"=w133, "error in"=w113) -> ("error out"=w112:errorcluster)  [unwired: 13 out]
      n178 = call <vilib>:"DAQmx Clear Task.vi"("task in"=w134, "error in"=w112) -> ("error out"=w100:errorcluster)  [unwired: 13 out]
      n179 = Merge Errors(w100, w99) -> (w101:errorcluster)
      "error out" <- w101
      n180 = call <vilib>:"General Error Handler.vi"("error in (no error)"=w101) -> ()  [unwired: 10 in, 5 out]
    }
    frame #2 {
      n181 = local read "Sweep enabled"() -> (w356:bool)
      n182 = case shown="True" w356 {
        frame False {
        }
        frame True {
          n183 = local read "Shutter Drive"() -> (w380:tag)
          n184 = call-poly <vilib>:"DAQmx Create Virtual Channel.vi"("physical channels"=w380) -> ("task out"=w379:refnum<k21>, "error out"=w378:errorcluster)  [unwired: 13 in]
          n185 = call-poly <vilib>:"DAQmx Write.vi"("task/channels in"=w379, "data"=dbl[] [0.0, 0.0, 0.0, 0.0], "error in"=w378) -> ("task out"=w381:refnum<k21>, "error out"=w382:errorcluster)  [unwired: 1 in, 10 out]
          n186 = call <vilib>:"DAQmx Clear Task.vi"("task in"=w381, "error in"=w382) -> ()  [unwired: 13 in, 1 out]
        }
      }
      n187 = case shown="False" "Spot" {
        frame False {
          n188 = local read "Machine Type"() -> (w361:u8)
          n189 = case shown="2" w361 {
            frame 0, Default {
            }
            frame 1 {
              w368 = TRUE ("Initialization")
              n190 = local read "COM port"() -> (w362:refnum<visa-resource-name>)
              n191 = call "FIB mode.vi"("Initialization"=w368, "FIB mode"=T5."SEM", "COM port in"=w362) -> ("COM port out"=w363:refnum<visa-resource-name>)  [unwired: 7 in, 1 out]
              n192 = call "Remcon32 command.vi"("SEM command"="edx 0", "COM port in"=w363) -> ("COM port out"=w364:refnum<visa-resource-name>)  [unwired: 6 in, 3 out]
              n193 = call "Remcon32 command.vi"("Close session"=w368, "SEM command"="frez", "COM port in"=w364) -> ()  [unwired: 5 in, 4 out]
            }
            frame 2 {
              n194 = local read "ActiveX Container"() -> (w373:refnum<k7>)
              n195 = call "SmartSEM Remote API set float.vi"("vValue"=sgl 2.0, "lpszParam"="DP_FIB_BLANKER_MODE" ("lpszCommand"), "ActiveX Container"=w373) -> ("error out"=w369:errorcluster, "reference out"=w370:refnum<k7>)  [unwired: 7 in]
              n196 = call "SmartSEM Remote API FIB mode.vi"("error in"=w369, "FIB mode"=T6."SEM", "ActiveX Container"=w370) -> ("error out"=w374:errorcluster, "reference out"=w375:refnum<k7>)  [unwired: 7 in]
              n197 = invoke class="_EMApi" method="Execute"(reference=w375, error in=w374, "lpszCommand"="CMD_FREEZE_ALL") -> ()  [unwired: 1 in, 4 out]
            }
          }
        }
        frame True {
        }
      }
      n198 = local read "Beam blank"() -> (w359:tag)
      n199 = local read "Ext scan"() -> (w358:tag)
      n200 = local read "ActiveX Container"() -> (w354:refnum<k7>)
      n201 = call "FIB beam blank.vi"("ActiveX Container"=w354, "Beam blanked"=TRUE, "lines"=w359) -> ()  [unwired: 2 in, 1 out]
      n202 = call "FIB ext scan.vi"("Ext on"=FALSE ("data"), "FIB Ext Scan"=w358) -> ()  [unwired: 9 in, 1 out]
    }
    frame #3 {
      n203 = local write "stop"(FALSE ("stop")) -> ()
      n204 = Request Deallocation(TRUE ("flag")) -> ()
    }
  }
